vi "Is Nested.vi"(10 "Alias":string, 11 "jettl Queue Actor in":refnum<class "jettl Queue Actor.lvclass">) -> (2 "Nested?":bool)   [LabVIEW 2021, in "jettl.lvlib" / "jettl Queue Actor.lvlib" / "jettl Queue Actor.lvclass"]
uses:
  jettl Queue Actor.lvclass
  jettl Queue Actor.lvclass/jettl Queue Actor.ctl
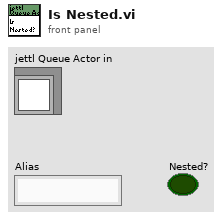
[diagram p1: front panel]
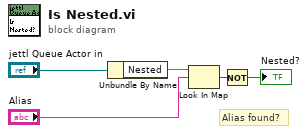
[diagram p0: block diagram]
diagram:
  # "Alias found?"
  n1 = Unbundle By Name("jettl Queue Actor in") -> ("Nested"=w4:map{string, refnum<data-value>})
  n2 = Look In Map(map=w4, key="Alias") -> (key not found?=w1:bool)  [unwired: 1 in, 1 out]
  n3 = Not(x=w1) -> (.not. x?=→"Nested?":bool)
